vi "programa 3.vi"() -> ()   [LabVIEW 2011]
panel:
  out "Observacion":string
  out "Boolean":bool
  in  "Numero":dbl
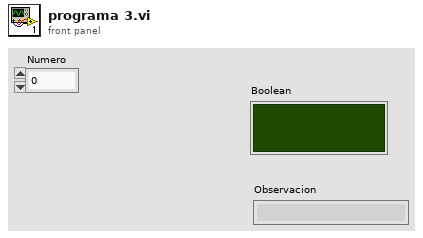
[diagram p1: front panel]
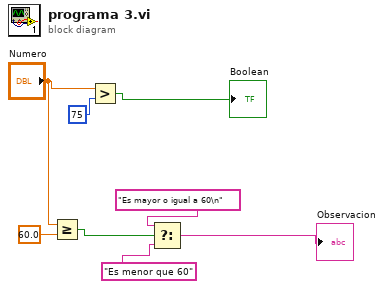
[diagram p0: block diagram]
diagram:
  n1 = Greater Or Equal?(x="Numero", y=60.0) -> (x >= y?=w4:bool)
  n2 = Greater?(x="Numero", y=75) -> (0:→"Boolean":bool)
  n3 = Select(t="Es mayor o igual a 60\n", s=w4, f="Es menor que 60") -> (s? t:f=→"Observacion":string)
